vi "GetWaveformByBusName(NoReorder).vi"(8 "error in (no error)":errorcluster, 10 "Bus Name":string, 11 "Acq Waveforms":waveform(sgl)[](array[waveform])) -> (0 "error out":errorcluster, 2 "Waveform of Bus":waveform(dbl)[](array[waveform]), 3 "Acq Waveforms Out":waveform(sgl)[](array[waveform]))   [LabVIEW 2017, in "McsaUtilities.lvlib"]
uses:
  <vilib>/addons/InsightCM/Utilities/MCSA/McsaUtilities.lvlib
  <vilib>/addons/InsightCM/Utilities/Analysis/MCSA/McsaAnalysisFunctions.lvlib
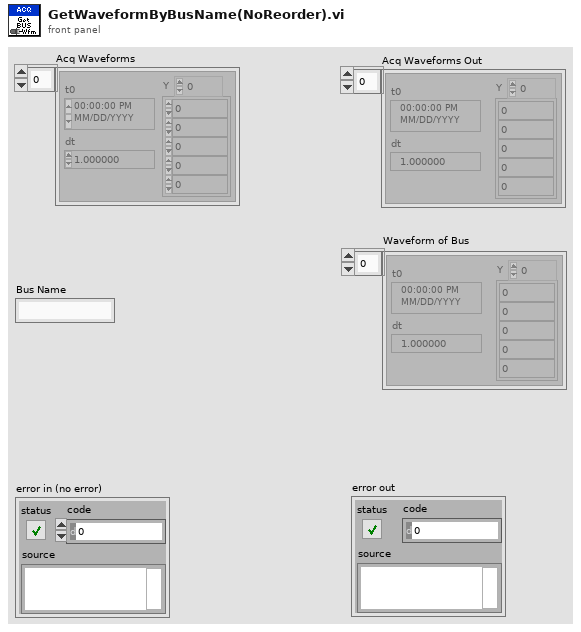
[diagram p1: front panel]
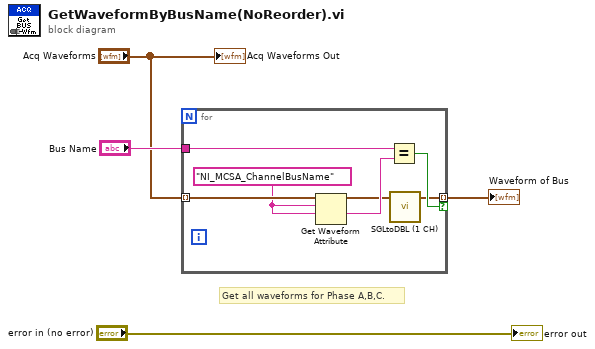
[diagram p0: block diagram]
diagram:
  # "Get all waveforms for Phase A,B,C."
  n1 = for {
    tunnel: "Acq Waveforms" -> [w11] mode=indexing
    tunnel: "Bus Name" -> [w10]
    tunnel: [w5] -> w1 mode=indexing if=w7
    w9 = "NI_MCSA_ChannelBusName" ("name")
    n2 = Get Waveform Attribute(5:w9, 6:w9, 7:w11) -> (1:w8:string, 3:w6:waveform(sgl))  [unwired: 1 in, 2 out]
    n3 = Equal?(x=w10, y=w8) -> (x = y?=w7:bool)
    n4 = call <vilib>:"SGLtoDBL (1 CH).vi"("Waveform in"=w6) -> ("Waveform out"=w5:waveform(dbl))  [unwired: 10 in]
  }
  "Waveform of Bus" <- w1
  "Acq Waveforms Out" <- "Acq Waveforms"
  "error out" <- "error in (no error)"
